vi "Q -- check range.vi"(4 "upper":dbl=99.0, 6 "lower":dbl, 11 "number":dbl=11.0) -> (0 "below ?":bool=TRUE, 1 "in range?":bool=TRUE, 2 "above ?":bool=TRUE, 3 "number in range":dbl, 5 "not a number?":bool=TRUE)   [LabVIEW 2015]
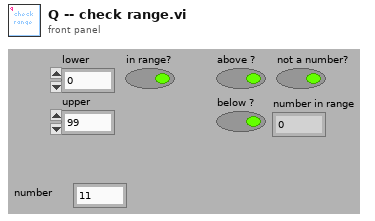
[diagram p1: front panel]
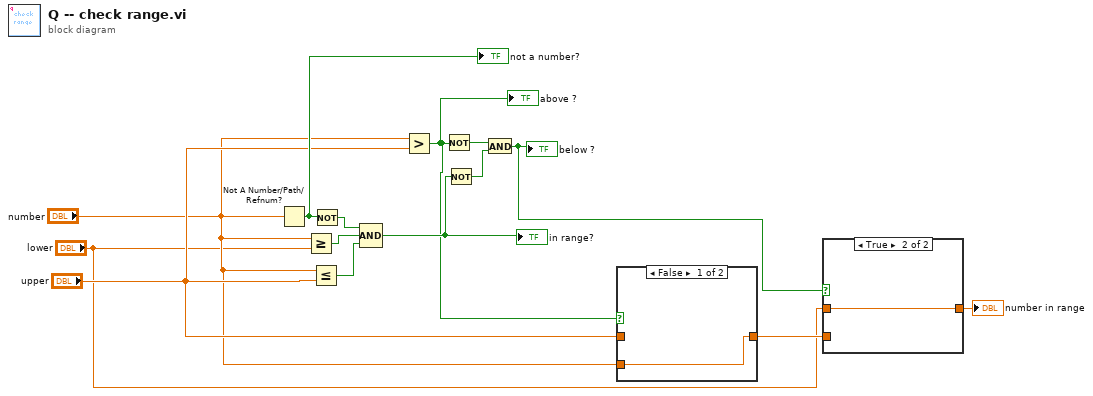
[diagram p0: block diagram]
diagram:
  n1 = Not A Number/Path/Refnum?(number/path/refnum="number") -> (NaN/Path/Refnum?=w9:bool)
  "not a number?" <- w9
  n2 = Greater Or Equal?(x="number", y="lower") -> (x >= y?=w13:bool)
  n3 = Less Or Equal?(x="number", y="upper") -> (x <= y?=w12:bool)
  n4 = Not(x=w9) -> (.not. x?=w14:bool)
  n5 = Compound Arithmetic op=AND(w14, w13, w12) -> (w8:bool)
  "in range?" <- w8
  n6 = Greater?(x="number", y="upper") -> (0:w7:bool)
  "above ?" <- w7
  n7 = Not(x=w7) -> (.not. x?=w11:bool)
  n8 = Not(x=w8) -> (.not. x?=w10:bool)
  n9 = And(x=w11, y=w10) -> (x .and. y?=w4:bool)
  "below ?" <- w4
  n10 = case shown="False" w7 {
    tunnel: [w15 w16] -> w3
    tunnel: "upper" -> [_ w16]
    tunnel: "number" -> [w15 _]
    frame False {
    }
    frame True {
    }
  }
  n11 = case shown="True" w4 {
    tunnel: [w17 w18] -> w1
    tunnel: "lower" -> [_ w18]
    tunnel: w3 -> [w17 _]
    frame False {
    }
    frame True {
    }
  }
  "number in range" <- w1
